vi "Master on RT Target.vi"() -> ()   [LabVIEW 2021]
doc: "Demonstrates how to use Modbus functions on RT to create a Modbus master communicating with a Modbus slave. It displays an array that shows the value of input registers on the slave and the value is updated every 1 second automatically."
uses:
  Modbus_v121c/API/Wrapper/Create TCP Master.vi
  Modbus_v121c/API/Master/Modbus Master.lvclass
  Modbus_v121c/API/Wrapper/API Main.lvlib
panel:
  in  "Stop":bool
  out "Input Registers":u16[](array[numeric])
  # "Overview: Demonstrates the use of the Modbus Master VIs on a LabVIEW Real-Time target to create a Modbus master and use the Modbus master to read the values of input registers from a Modbus slave every one second.\nRequirements: LabVIEW Real-Time Module\nInstructions:\n1. Ensure Slave On RT Target.vi is already running.\n2. Run the VI.\n3. Click Stop to stop the VI."
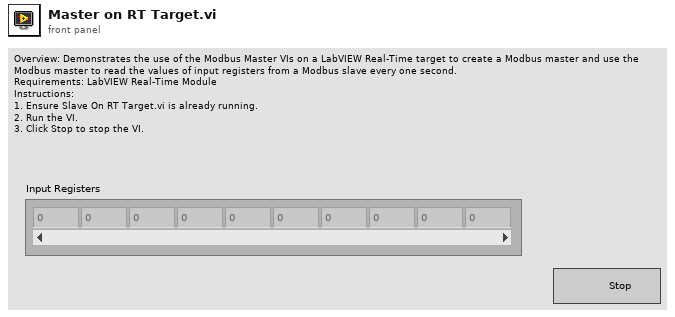
[diagram p1: front panel]
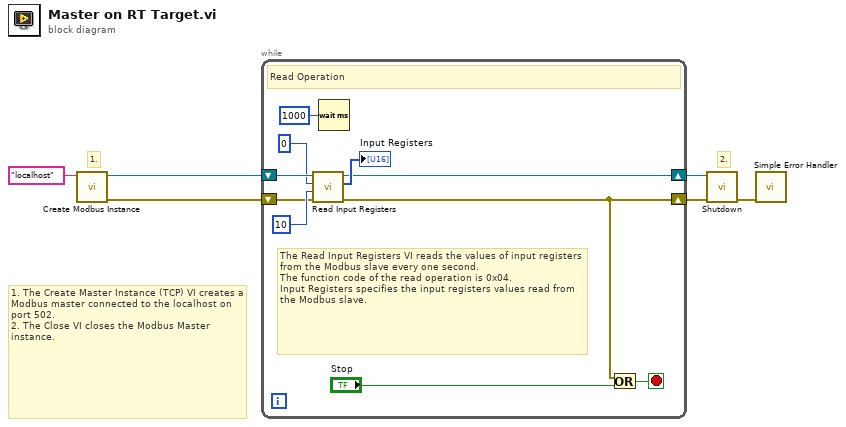
[diagram p0: block diagram]
diagram:
  # "2."
  # "1."
  # "1. The Create Master Instance (TCP) VI creates a Modbus master connected to the localhost on port 502.\n2. The Close VI closes the Modbus Master instance."
  n1 = call-poly "Create Modbus Instance.vi"("address"="localhost") -> ("error out"=w4:errorcluster, "TCP master instance"=w5:refnum<class "Modbus Master.lvclass">)  [unwired: 9 in]
  n2 = while {
    shift-right: [w9] -> w3
    shift-left: w4 -> [w13]
    shift-right: [w10] -> w2
    shift-left: w5 -> [w14]
    stop <- w8 stop-if-true
    # "The Read Input Registers VI reads the values of input registers from the Modbus slave every one second.\nThe function code of the read operation is 0x04.\nInput Registers specifies the input registers values read from the Modbus slave."
    # "Read Operation"
    n3 = call-dynamic "Read Input Registers.vi"("error in (no error)"=w13, "number of input registers"=u16 10 ("number of inputs"), "starting address"=u16 0, "Modbus master in"=w14) -> ("error out"=w9:errorcluster, "register values"=→"Input Registers":u16[], "Modbus master out"=w10:refnum<class "Modbus Master.lvclass">)  [unwired: 5 in]
    n4 = Wait (ms)(milliseconds to wait=u32 1000) -> ()  [unwired: 1 out]
    n5 = Or(x=w9, y="Stop") -> (x .or. y?=w8:bool)
  }
  n6 = call-dynamic "Shutdown.vi"("error in (no error)"=w3, "Modbus master in"=w2) -> ("error out"=w1:errorcluster)  [unwired: 9 in]
  n7 = call <vilib>:"Simple Error Handler.vi"("error in (no error)"=w1) -> ()  [unwired: 4 in, 5 out]
